vi "Set_Validation.vi"(0 "GPIB address":string, 3 "error in (no error)":errorcluster) -> (7 "error out":errorcluster)   [LabVIEW 2010]
panel:
  out "data Out":string
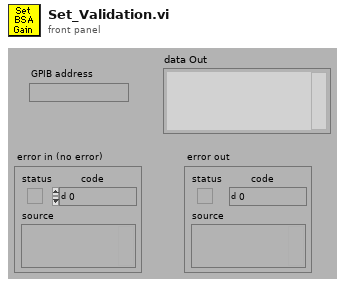
[diagram p1: front panel]
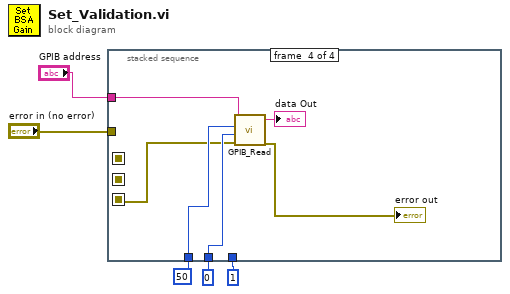
[diagram p0: block diagram]
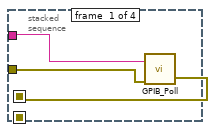
[diagram p2: hidden frame]
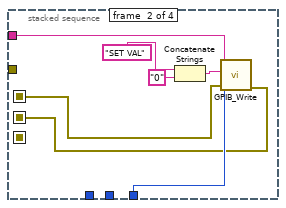
[diagram p3: hidden frame]
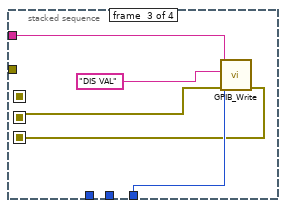
[diagram p4: hidden frame]
diagram:
  n1 = stacked-sequence {
    seq-local: [w6 _ _ _] -> [_ w11 _ _]
    seq-local: [_ w10 _ _] -> [_ _ w17 _]
    seq-local: [_ _ w16 _] -> [_ _ _ w23]
    tunnel: "GPIB address" -> [w8 w15 w20 w26]
    tunnel: 1 -> [_ w14 w19 _]
    tunnel: 0 -> [_ _ _ w25]
    tunnel: 50 -> [_ _ _ w24]
    tunnel: "error in (no error)" -> [w7 _ _ _]
    frame #0 {
      n2 = call "GPIB_Poll.vi"("error in"=w7, "address string"=w8) -> ("error out"=w6:errorcluster)  [unwired: 1 out]
    }
    frame #1 {
      n3 = Concatenate Strings("SET VAL", "0" ("string")) -> (w12:string)
      n4 = call "GPIB_Write.vi"("address string"=w15, "data In"=w12, "mode (0)"=w14, "error in"=w11) -> ("error out"=w10:errorcluster)  [unwired: 1 in, 1 out]
    }
    frame #2 {
      n5 = call "GPIB_Write.vi"("address string"=w20, "data In"="DIS VAL", "mode (0)"=w19, "error in"=w17) -> ("error out"=w16:errorcluster)  [unwired: 1 in, 1 out]
    }
    frame #3 {
      n6 = call "GPIB_Read.vi"("address string"=w26, "byte count"=w24, "mode (0)"=w25, "error in"=w23) -> ("data Out"=→"data Out":string, "error out"=→"error out":errorcluster)  [unwired: 1 in, 1 out]
    }
  }
